vi "Varian_PUMP_START.vi"(5 "APX:APITurbo_START":bool, 7 "PV Name":string, 8 "error in":errorcluster, 10 "APX:AP1TurboF":dbl, 11 "VISA Refnum in":refnum<visa-resource-name>) -> (0 "error out":errorcluster, 3 "VISA Refnum out":refnum<visa-resource-name>)   [LabVIEW 2015]
uses:
  <userlib>/caLab/Private/Put_DBL_PV.vi
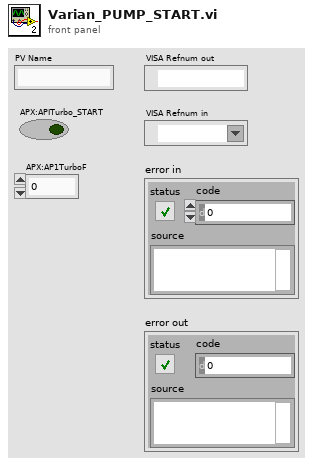
[diagram p1: front panel]
types:
  T1 = enum16{"START", "STOP", "REMOTE/SERIAL", "REMOTE", "SERIAL", "START/STOP", "PUMP STATUS", "Driving Frequency", "PUMP POWER", "PRESSURE"}
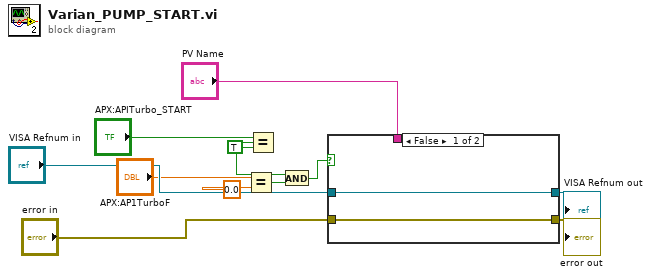
[diagram p0: block diagram]
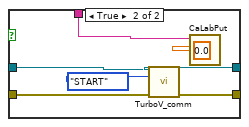
[diagram p2: hidden frame]
diagram:
  n1 = Equal?(x="APX:AP1TurboF", y=0.0) -> (x = y?=w1:bool)
  n2 = Equal?(x="APX:APITurbo_START", y=TRUE) -> (x = y?=w2:bool)
  n3 = And(x=w2, y=w1) -> (x .and. y?=w7:bool)
  n4 = case shown="False" w7 {
    tunnel: [w14 w20] -> w10
    tunnel: [w13 w19] -> w11
    tunnel: "VISA Refnum in" -> [w14 w18]
    tunnel: "error in" -> [w13 w17]
    tunnel: "PV Name" -> [_ w15]
    frame False {
    }
    frame True {
      n5 = call "TurboV_comm.vi"("VISA resource name"=w18, "Command"=T1."START", "error in (no error)"=w17) -> ("VISA resource name out"=w20:refnum<visa-resource-name>, "error out"=w19:errorcluster)  [unwired: 10 in, 1 out]
      n6 = call-poly <userlib>:"CaLabPut.vi"("Value"=0.0, "PV Name"=w15) -> ()  [unwired: 6 in, 4 out]
    }
  }
  "error out" <- w11
  "VISA Refnum out" <- w10
